vi "Any string array items in string.vi"(8 "error in (no error)":errorcluster, 9 "Ignore case (n)":bool, 10 "Strings to look for":string[](array[string]), 11 "String buffer":string) -> (0 "error out":errorcluster, 3 "In string?":bool)   [LabVIEW 2024]
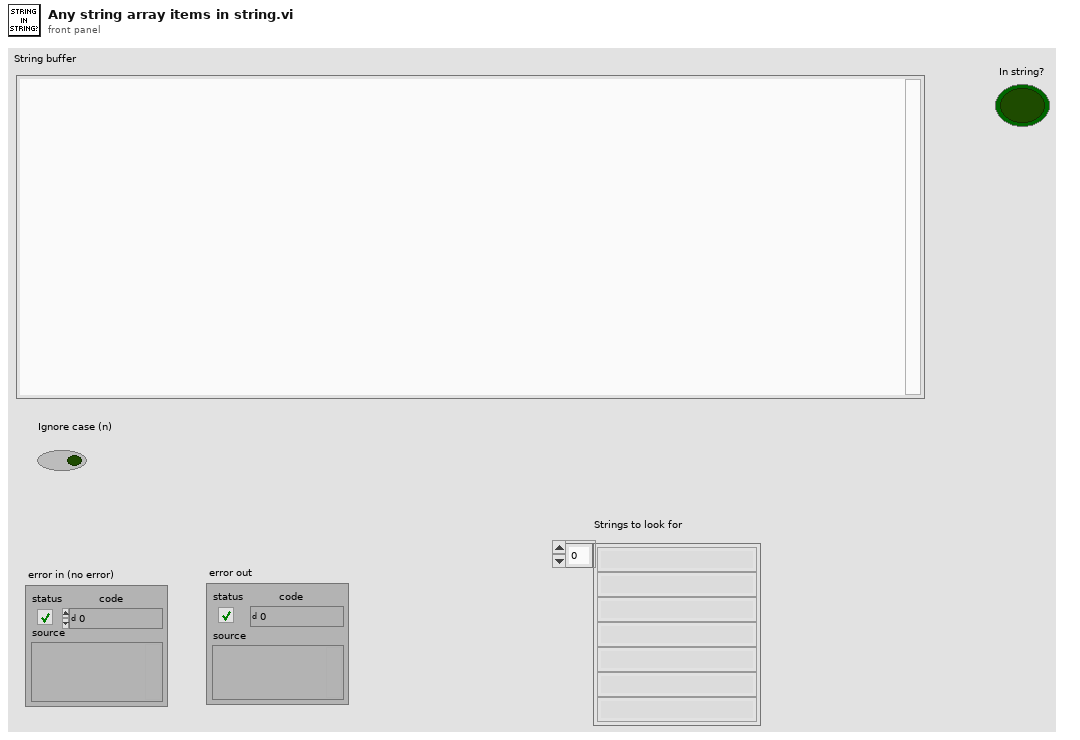
[diagram p1: front panel]
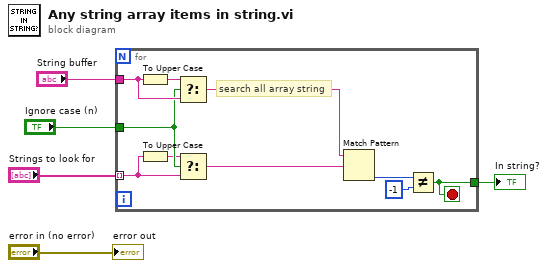
[diagram p0: block diagram]
diagram:
  n1 = for {
    tunnel: "String buffer" -> [w11]
    tunnel: "Strings to look for" -> [w6] mode=indexing
    tunnel: [w13] -> w2
    tunnel: "Ignore case (n)" -> [w10]
    stop <- w13 stop-if-true
    # "search all array string"
    n2 = To Upper Case(1:w11) -> (0:w12:string)
    n3 = To Upper Case(1:w6) -> (0:w9:string)
    n4 = Select(t=w12, s=w10, f=w11) -> (s? t:f=w7:string)
    n5 = Select(t=w9, s=w10, f=w6) -> (s? t:f=w8:string)
    n6 = Match Pattern(string=w7, regular expression=w8) -> (offset past match=w14:i32)  [unwired: 1 in, 3 out]
    n7 = Not Equal?(x=w14, y=-1) -> (x != y?=w13:bool)
  }
  "In string?" <- w2
  "error out" <- "error in (no error)"
